vi "KE26XX Real Converter Usage.vi"(4 "Limit (0.01 A)":dbl=0.01, 5 "Measure Count (10)":u32=10, 6 "Level (5 V)":dbl=5.0, 7 "Error Query (False)":bool, 8 "error in (no error)":errorcluster, 11 "VISA resource name":refnum<visa-resource-name>) -> (0 "error out":errorcluster, 2 "Data Array Out":sgl[](array[numeric]))   [LabVIEW 2009]
doc: "This example demonstrates how to retreive Real 64 data from the instrument and how to use the Real 64 Converter VI to convert this data into an array of doubles.\n\nThis example demonstrates the following:\n• Clearing and configuring a non-volatile reading buffer\n• Quickly seting up the source\n• Quickly configuring the measure hardware\n• Take measurements into a reading buffer\n• Configure the data output format\n• Print back a reading buffer\n• Convert the returned data into an array of doubles"
uses:
  <instrlib>/Keithley 2600 Series/Public/Channel.ctl
  <instrlib>/Keithley 2600 Series/Keithley 2600 Series.lvlib
panel:
  # "(c) 2008 Keithley Instruments, Inc.  ALL RIGHTS RESERVED."
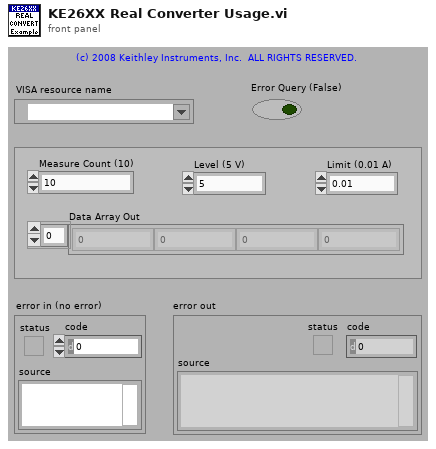
[diagram p1: front panel]
types:
  T1 = enum32{"Normal", "Big Endian", "Little Endian", "Network", "Swapped"}
  T2 = enum32{"ASCII", "Real 32", "Real 64", "Single Precision Real", "Double Precision Real"}
  T3 = enum32{"Current", "Voltage", "IV", "Resistance", "Power"}
  T4 = typedef "Keithley 2600 Series.lvlib/Channel.ctl" = enum32{"Channel A", "Channel B"}
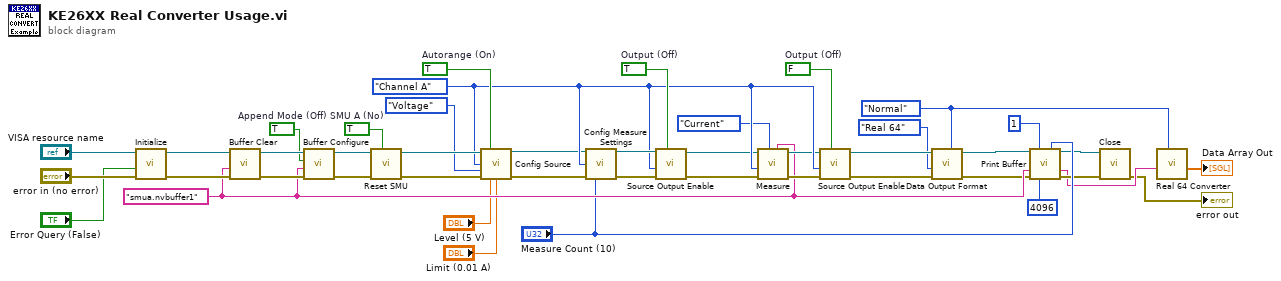
[diagram p0: block diagram]
diagram:
  w7 = T1."Normal" ("Byte Order (Normal)")
  w22 = FALSE  # Output (Off)
  w30 = TRUE  # Output (Off)
  w33 = TRUE  # Autorange (On)
  w29 = Channel."Channel A" ("Channel (Channel A)")
  w37 = TRUE  # SMU A (No)
  w40 = TRUE  # Append Mode (Off)
  w20 = "smua.nvbuffer1" ("Buffer Name")
  n1 = call <instrlib>:"Initialize.vi"("error in (no error)"="error in (no error)", "Error Query (False)"="Error Query (False)", "VISA resource name"="VISA resource name") -> ("error out"=w43:errorcluster, "VISA resource name out"=w44:refnum<visa-resource-name>)  [unwired: 3 in, 4 out]
  n2 = call <instrlib>:"Buffer Clear.vi"("error in (no error)"=w43, "Buffer Name"=w20, "VISA resource name"=w44) -> ("error out"=w41:errorcluster, "VISA resource name out"=w42:refnum<visa-resource-name>)  [unwired: 7 out]
  n3 = call <instrlib>:"Buffer Configure.vi"("error in (no error)"=w41, "Buffer Name"=w20, "Append Mode (Off)"=w40, "VISA resource name"=w42) -> ("error out"=w38:errorcluster, "VISA resource name out"=w39:refnum<visa-resource-name>)  [unwired: 3 in, 3 out]
  n4 = call <instrlib>:"Reset SMU.vi"("SMU A (No)"=w37, "error in (no error)"=w38, "VISA resource name"=w39) -> ("error out"=w35:errorcluster, "VISA resource name out"=w36:refnum<visa-resource-name>)  [unwired: 2 in, 5 out]
  n5 = call <instrlib>:"Config Source.vi"("VISA resource name"=w36, "Autorange (On)"=w33, "Channel (Channel A)"=w29, "Function (Current)"=enum32{"Current", "Voltage"}."Voltage", "error in"=w35, "Level (0.000)"="Level (5 V)", "Limit (0.1)"="Limit (0.01 A)") -> ("VISA resource name out"=w24:refnum<visa-resource-name>, "error out"=w23:errorcluster)  [unwired: 4 in, 3 out]
  n6 = call <instrlib>:"Config Measure Settings.vi"("VISA resource name"=w24, "Channel (Channel A)"=w29, "error in"=w23, "Measure Count (1)"="Measure Count (10)") -> ("VISA resource name out"=w32:refnum<visa-resource-name>, "error out"=w31:errorcluster)  [unwired: 6 in, 4 out]
  n7 = call <instrlib>:"Source Output Enable.vi"("Output (Off)"=w30, "error in (no error)"=w31, "Channel (Channel A)"=w29, "VISA resource name"=w32) -> ("error out"=w28:errorcluster, "VISA resource name out"=w27:refnum<visa-resource-name>)  [unwired: 1 in, 5 out]
  n8 = call <instrlib>:"Measure.vi"("Buffer 1"=w20, "Function (Current)"=T3."Current", "error in (no error)"=w28, "Channel (Channel A)"=w29, "VISA resource name"=w27) -> ("error out"=w25:errorcluster, "VISA resource name out"=w26:refnum<visa-resource-name>)  [unwired: 2 in, 3 out]
  n9 = call <instrlib>:"Source Output Enable.vi"("Output (Off)"=w22, "error in (no error)"=w25, "Channel (Channel A)"=w29, "VISA resource name"=w26) -> ("error out"=w11:errorcluster, "VISA resource name out"=w12:refnum<visa-resource-name>)  [unwired: 1 in, 5 out]
  n10 = call <instrlib>:"Data Output Format.vi"("Byte Order (Normal)"=w7, "error in (no error)"=w11, "Data Format (ASCII)"=T2."Real 64", "VISA resource name"=w12) -> ("error out"=w9:errorcluster, "VISA resource name out"=w8:refnum<visa-resource-name>)  [unwired: 2 in, 4 out]
  n11 = call <instrlib>:"Print Buffer.vi"("VISA resource name"=w8, "Start Index (1)"=u32 1, "End Index (1)"="Measure Count (10)", "Buffer Name(s)"=w20, "error in (no error)"=w9, "Byte Count (1024)"=u32 4096) -> ("VISA resource name out"=w16:refnum<visa-resource-name>, "Buffer Data"=w14:string, "error out"=w17:errorcluster)  [unwired: 1 in, 6 out]
  n12 = call <instrlib>:"Close.vi"("error in (no error)"=w17, "VISA resource name"=w16) -> ("error out"=→"error out":errorcluster)  [unwired: 9 out]
  n13 = call <instrlib>:"Real 64 Converter.vi"("Byte Order (Normal)"=w7, "Data In"=w14) -> ("Data Array Out"=→"Data Array Out":dbl[])  [unwired: 9 out]
